vi "midi_in.device_name.get.vi"(8 "error in (no error)":errorcluster, 10 "device_index":i32, 11 "LabVIEW-MIDI-XPLAT in":refnum<class "LabVIEW-MIDI-XPLAT.lvclass">) -> (0 "error out":errorcluster, 2 "buffer":string, 3 "LabVIEW-MIDI-XPLAT out":refnum<class "LabVIEW-MIDI-XPLAT.lvclass">, 4 "Return":i32)   [LabVIEW 2020, in "LabVIEW-MIDI-XPLAT.lvclass"]
uses:
  LabVIEW-MIDI-XPLAT.lvclass
  LabVIEW-MIDI-XPLAT.lvclass/LabVIEW-MIDI-XPLAT.ctl
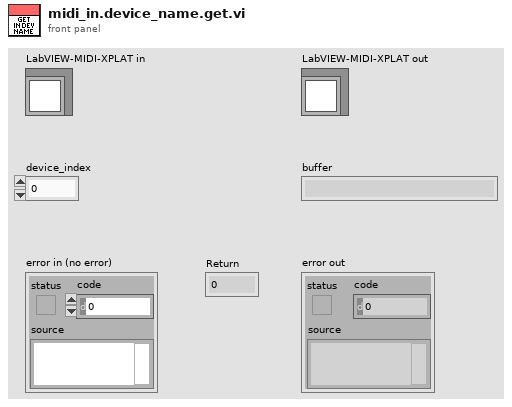
[diagram p1: front panel]
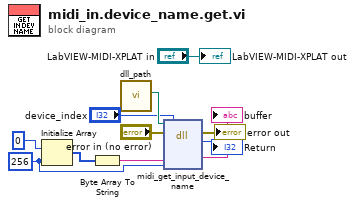
[diagram p0: block diagram]
diagram:
  w6 = 256 ("dimension size")
  n1 = Initialize Array(u8 0, w6) -> (w4:u8[])
  n2 = Byte Array To String(unsigned byte array=w4) -> (string=w7:string)
  n3 = call "dll_path.vi"() -> ("dll"=w8:path)  [unwired: 11 in]
  n4 = dll-call lib="C:/code/LabVIEW-MIDI-XPLAT/dist/TomMIDIllan_*.*" fn="midi_get_input_device_name"(path in=w8, error in="error in (no error)", "device_index"="device_index", "buffer"=w7, "buffer_size"=w6) -> (error out=→"error out":errorcluster, "Return"=→"Return":i32, "buffer"=→"buffer":string)  [unwired: 3 in, 1 out]
  "LabVIEW-MIDI-XPLAT out" <- "LabVIEW-MIDI-XPLAT in"
